vi "SettingDigitalOutDemo.vi"   [LabVIEW 2016]
doc: "This VI demonstrates how to adjust digital out signals and how to filter certain types of signals (here: digital out signals)."
types:
  T1 = cluster{"Devices":refnum<k24>[], "Signals":refnum<k24>[]}
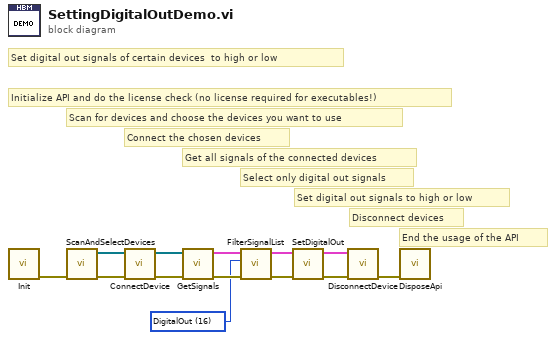
[diagram p0: block diagram]
diagram:
  w4 = 16 items=["Measurable"=1, "AnalogIn"=2, "AnalogOut"=4, "DigitalIn"=8, "DigitalOut"=16, "Virtual"=32] ("SignalTypeToFilter")
  # "Disconnect devices"
  # "End the usage of the API"
  # "Set digital out signals to high or low"
  # "Set digital out signals of certain devices  to high or low"
  # "Select only digital out signals"
  # "Get all signals of the connected devices"
  # "Connect the chosen devices"
  # "Scan for devices and choose the devices you want to use"
  # "Initialize API and do the license check (no license required for executables!)"
  n1 = call "Init.vi"() -> ("Error out"=w9:errorcluster)  [unwired: 8 in, 2 out]
  n2 = call "ScanAndSelectDevices.vi"("Error in"=w9) -> ("Error out"=w13:errorcluster, "SelectedDevices"=w11:refnum<k24>[])  [unwired: 8 in, 1 out]
  n3 = call "ConnectDevice.vi"("Error in"=w13, "Devices"=w11) -> ("Error out"=w12:errorcluster, "Devices"=w10:refnum<k24>[])  [unwired: 7 in, 1 out]
  n4 = call "GetSignals.vi"("Error in"=w12, "Devices"=w10) -> ("Error out"=w8:errorcluster, "DevicesAndSignals"=w7:T1)  [unwired: 7 in, 1 out]
  n5 = call "FilterSignalList.vi"("Error in"=w8, "SignalTypeToFilter"=w4, "DevicesAndSignals"=w7) -> ("Error out"=w5:errorcluster, "DevicesAndSignals"=w6:T1)  [unwired: 7 in]
  n6 = call "SetDigitalOut.vi"("Error in"=w5, "DevicesAndSignals"=w6) -> ("Error out"=w3:errorcluster, "DevicesAndSignals"=w1:T1)  [unwired: 8 in]
  n7 = call "DisconnectDevice.vi"("Error in"=w3, "DevicesAndSignals"=w1) -> ("Error out"=w2:errorcluster)  [unwired: 9 in]
  n8 = call "DisposeApi.vi"("Error in"=w2) -> ()  [unwired: 10 in, 1 out]
